vi "RF Filter Zero Phase.vi"(8 "Error In":errorcluster, 9 "RF Signals In":waveform(dbl)[](array[waveform])=[{"t0"=timestamp(9.964599999999664e-07 s since 1904-01-01), "dt"=9.99999993922529e-09, "Y"=array[502 elements]}], 10 "Filter Definition":T1={"Upper Cutoff [Hz]"=1000000.0, "Lower Cutoff [Hz]"=2000000.0, "Order"=1, "Type"=enum."Bandpass"} {"Upper Cutoff [Hz]" min=100000.0 max=100000000.0 step=100000.0 format="%#_6p"; "Lower Cutoff [Hz]" min=100000.0 max=100000000.0 step=100000.0 format="%#_6p"}) -> (0 "Error Out":errorcluster, 1 "Filtered RF Signals":waveform(dbl)[](array[waveform])=[{"t0"=timestamp(9.964599999999664e-07 s since 1904-01-01), "dt"=9.99999993922529e-09, "Y"=array[502 elements]}])   [LabVIEW 2019]
uses:
  RF Filter Control.ctl
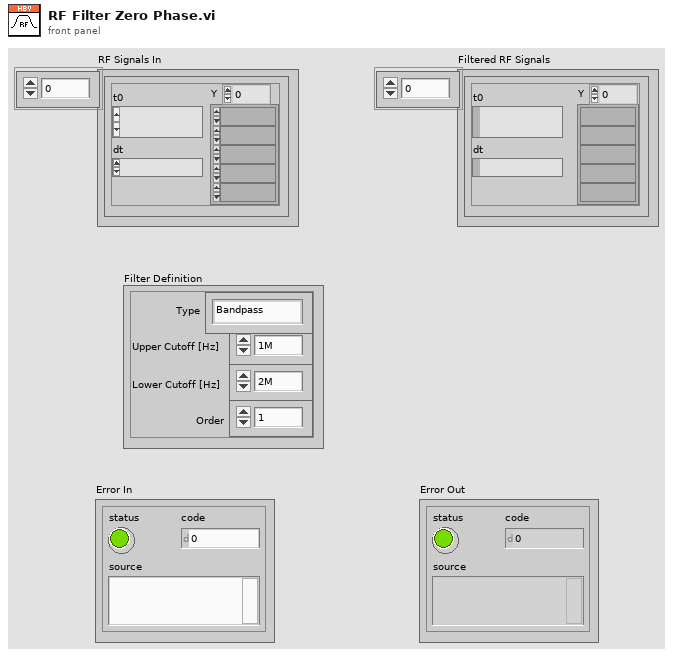
[diagram p1: front panel]
types:
  T1 = typedef "RF Filter Control.ctl" = cluster{"Upper Cutoff [Hz]":dbl, "Lower Cutoff [Hz]":dbl, "Order":i32, "Type":enum16{"Bandpass", "AC", "No Filter"}}
  T2 = cluster{"filter structure":enum32{"IIR 2nd Order", "IIR 4th Order"}, "Reverse Coefficients":dbl[], "Forward Coefficients":dbl[]}
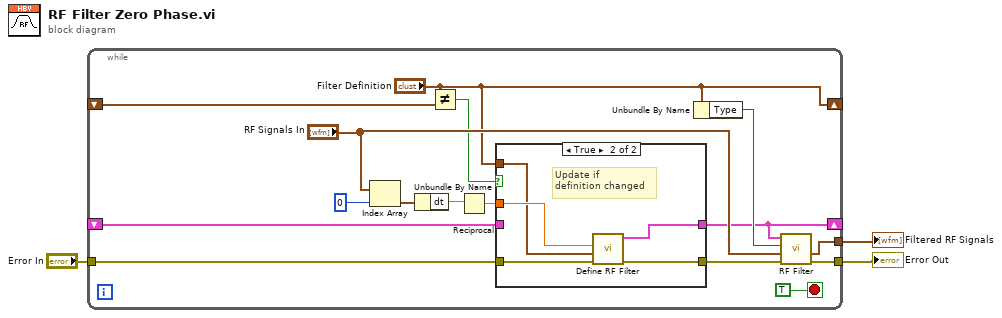
[diagram p0: block diagram]
diagram:
  n1 = while {
    tunnel: "Error In" -> [w17]
    tunnel: [w16] -> w1
    shift-right: [w7] -> _
    shift-left: _ -> [w4]
    shift-right: ["Filter Definition"] -> _
    shift-left: _ -> [w6]
    tunnel: [w18] -> w3
    stop <- TRUE stop-if-true
    n2 = Index Array(array="RF Signals In", index=0) -> (element=w14:waveform(dbl))
    n3 = Unbundle By Name(w14) -> ("dt"=w12:dbl)
    n4 = Not Equal?(x="Filter Definition", y=w6) -> (x != y?=w8:bool)
    n5 = Reciprocal(x=w12) -> (1/x=w11:dbl)
    n6 = case shown="True" w8 {
      tunnel: w17 -> [w21 w26]
      tunnel: [w21 w25] -> w9
      tunnel: w11 -> [_ w24]
      tunnel: [w20 w23] -> w7
      tunnel: "Filter Definition" -> [_ w22]
      tunnel: w4 -> [w20 _]
      frame False {
      }
      frame True {
        # "Update if \ndefinition changed"
        n7 = call "Define RF Filter.vi"("Error In"=w26, "Filter Definition"=w22, "Sample Rate [1/s]"=w24) -> ("Error Out"=w25:errorcluster, "IIR Filter Coefficients"=w23:T2)  [unwired: 7 in]
      }
    }
    n8 = Unbundle By Name("Filter Definition") -> ("Type"=w10:enum16{"Bandpass", "AC", "No Filter"})
    n9 = call "RF Filter.vi"("Error In"=w9, "RF Signals In"="RF Signals In", "Type"=w10, "IIR Filter Cluster in"=w7) -> ("Error Out"=w16:errorcluster, "Filtered Signals"=w18:waveform(dbl)[])  [unwired: 6 in]
  }
  "Error Out" <- w1
  "Filtered RF Signals" <- w3
